vi "Unrock_Cluster_To_Unrock_Data.vi"(0 "Unrock_Cluster":T2, 1 "NAM":string, 2 "TDN":string, 3 "PROD":string, 4 "CALD":string, 5 "REV":string) -> (17 "Cluster67":T1)   [LabVIEW 2019]
uses:
  Unrock_Cluster.ctl
  Test_load.ctl
  Hardness_test.ctl
  Unrock_Data.ctl
  TEST.lvclass
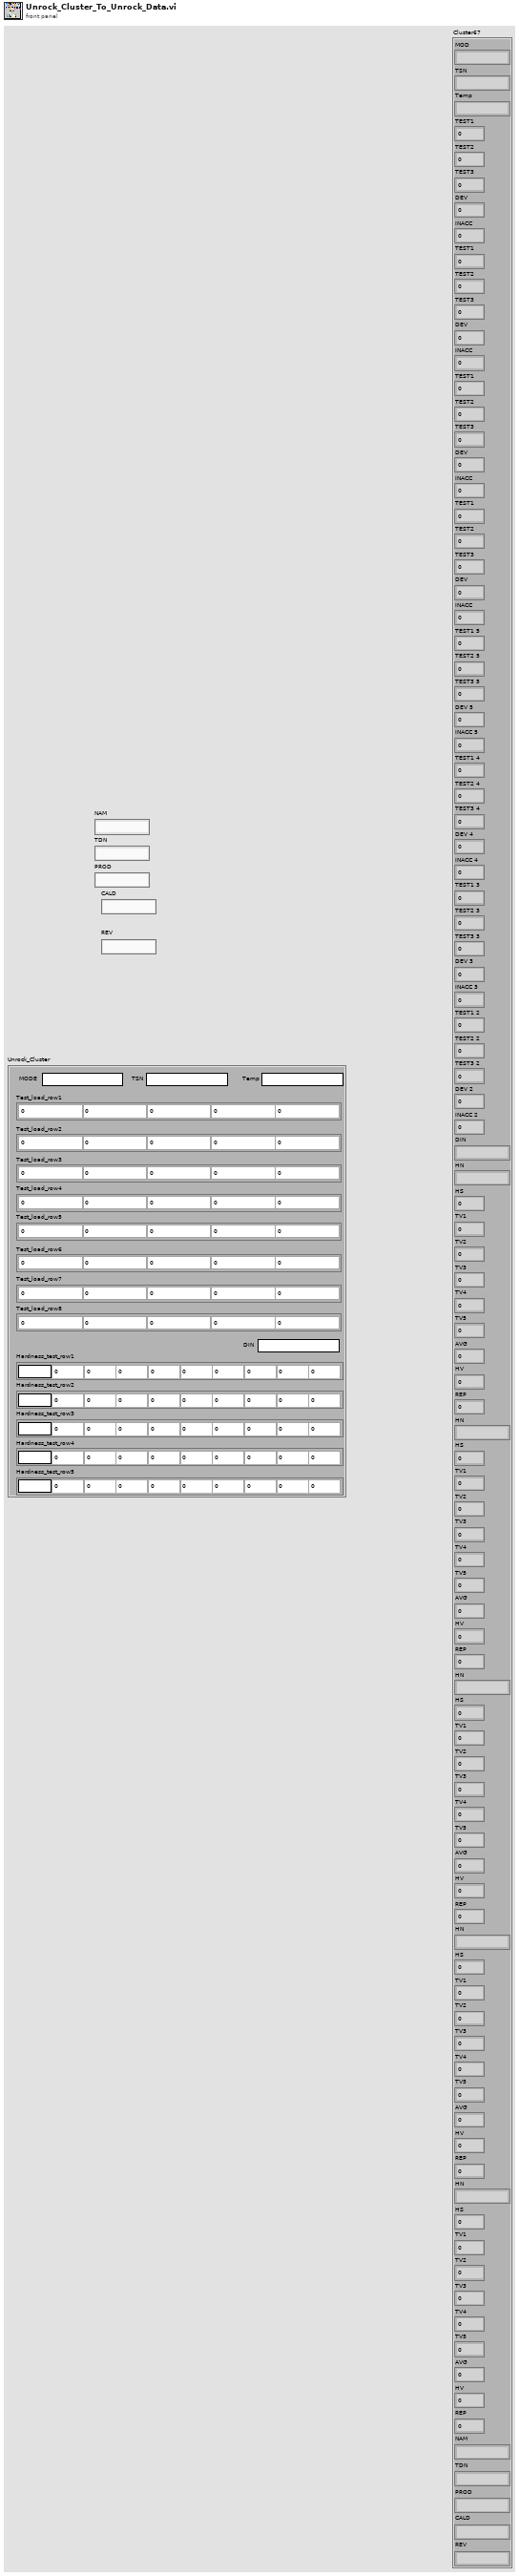
[diagram p1: front panel]
types:
  T1 = typedef "TEST.lvclass/Unrock_Data.ctl" = cluster{"MOD":string, "TSN":string, "Temp":string, "TEST1":sgl, "TEST2":sgl, "TEST3":sgl, "DEV":sgl, "INACC":sgl, "TEST1":sgl, "TEST2":sgl, "TEST3":sgl, "DEV":sgl, "INACC":sgl, "TEST1":sgl, "TEST2":sgl, "TEST3":sgl, "DEV":sgl, "INACC":sgl, "TEST1":sgl, "TEST2":sgl, "TEST3":sgl, "DEV":sgl, "INACC":sgl, "TEST1 5":sgl, "TEST2 5":sgl, "TEST3 5":sgl, "DEV 5":sgl, "INACC 5":sgl, "TEST1 4":sgl, "TEST2 4":sgl, "TEST3 4":sgl, "DEV 4":sgl, "INACC 4":sgl, "TEST1 3":sgl, "TEST2 3":sgl, "TEST3 3":sgl, "DEV 3":sgl, "INACC 3":sgl, "TEST1 2":sgl, "TEST2 2":sgl, "TEST3 2":sgl, "DEV 2":sgl, "INACC 2":sgl, "DIN":string, "HN":string, "HS":sgl, "TV1":sgl, "TV2":sgl, "TV3":sgl, "TV4":sgl, "TV5":sgl, "AVG":sgl, "HV":sgl, "REP":sgl, "HN":string, "HS":sgl, "TV1":sgl, "TV2":sgl, "TV3":sgl, "TV4":sgl, "TV5":sgl, "AVG":sgl, "HV":sgl, "REP":sgl, "HN":string, "HS":sgl, "TV1":sgl, "TV2":sgl, "TV3":sgl, "TV4":sgl, "TV5":sgl, "AVG":sgl, "HV":sgl, "REP":sgl, "HN":string, "HS":sgl, "TV1":sgl, "TV2":sgl, "TV3":sgl, "TV4":sgl, "TV5":sgl, "AVG":sgl, "HV":sgl, "REP":sgl, "HN":string, "HS":sgl, "TV1":sgl, "TV2":sgl, "TV3":sgl, "TV4":sgl, "TV5":sgl, "AVG":sgl, "HV":sgl, "REP":sgl, "NAM":string, "TDN":string, "PROD":string, "CALD":string, "REV":string}
  T2 = typedef "TEST.lvclass/Unrock_Cluster.ctl" = cluster{"MODE":string, "TSN":string, "Temp":string, "Test_load_row1":T3, "Test_load_row2":T3, "Test_load_row3":T3, "Test_load_row4":T3, "Test_load_row5":T3, "Test_load_row6":T3, "Test_load_row7":T3, "Test_load_row8":T3, "DIN":string, "Hardness_test_row1":T4, "Hardness_test_row2":T4, "Hardness_test_row3":T4, "Hardness_test_row4":T4, "Hardness_test_row5":T4}
  T3 = typedef "TEST.lvclass/Test_load.ctl" = cluster{"TEST1":sgl, "TEST2":sgl, "TEST3":sgl, "DEV":sgl, "INACC":sgl}
  T4 = typedef "TEST.lvclass/Hardness_test.ctl" = cluster{"HN":string, "HS":sgl, "TV1":sgl, "TV2":sgl, "TV3":sgl, "TV4":sgl, "TV5":sgl, "AVG":sgl, "HV":sgl, "REP":sgl}
  T5 = cluster{"MODE":string, "TSN":string, "Temp":string, "TEST1":sgl, "TEST2":sgl, "TEST3":sgl, "DEV":sgl, "INACC":sgl, "TEST1":sgl, "TEST2":sgl, "TEST3":sgl, "DEV":sgl, "INACC":sgl, "TEST1":sgl, "TEST2":sgl, "TEST3":sgl, "DEV":sgl, "INACC":sgl, "TEST1":sgl, "TEST2":sgl, "TEST3":sgl, "DEV":sgl, "INACC":sgl, "TEST1":sgl, "TEST2":sgl, "TEST3":sgl, "DEV":sgl, "INACC":sgl, "TEST1":sgl, "TEST2":sgl, "TEST3":sgl, "DEV":sgl, "INACC":sgl, "TEST1":sgl, "TEST2":sgl, "TEST3":sgl, "DEV":sgl, "INACC":sgl, "TEST1":sgl, "TEST2":sgl, "TEST3":sgl, "DEV":sgl, "INACC":sgl, "DIN":string, "HN":string, "HS":sgl, "TV1":sgl, "TV2":sgl, "TV3":sgl, "TV4":sgl, "TV5":sgl, "AVG":sgl, "HV":sgl, "REP":sgl, "HN":string, "HS":sgl, "TV1":sgl, "TV2":sgl, "TV3":sgl, "TV4":sgl, "TV5":sgl, "AVG":sgl, "HV":sgl, "REP":sgl, "HN":string, "HS":sgl, "TV1":sgl, "TV2":sgl, "TV3":sgl, "TV4":sgl, "TV5":sgl, "AVG":sgl, "HV":sgl, "REP":sgl, "HN":string, "HS":sgl, "TV1":sgl, "TV2":sgl, "TV3":sgl, "TV4":sgl, "TV5":sgl, "AVG":sgl, "HV":sgl, "REP":sgl, "HN":string, "HS":sgl, "TV1":sgl, "TV2":sgl, "TV3":sgl, "TV4":sgl, "TV5":sgl, "AVG":sgl, "HV":sgl, "REP":sgl, "NAM":string, "TDN":string, "PROD":string, "CALD":string, "REV":string}
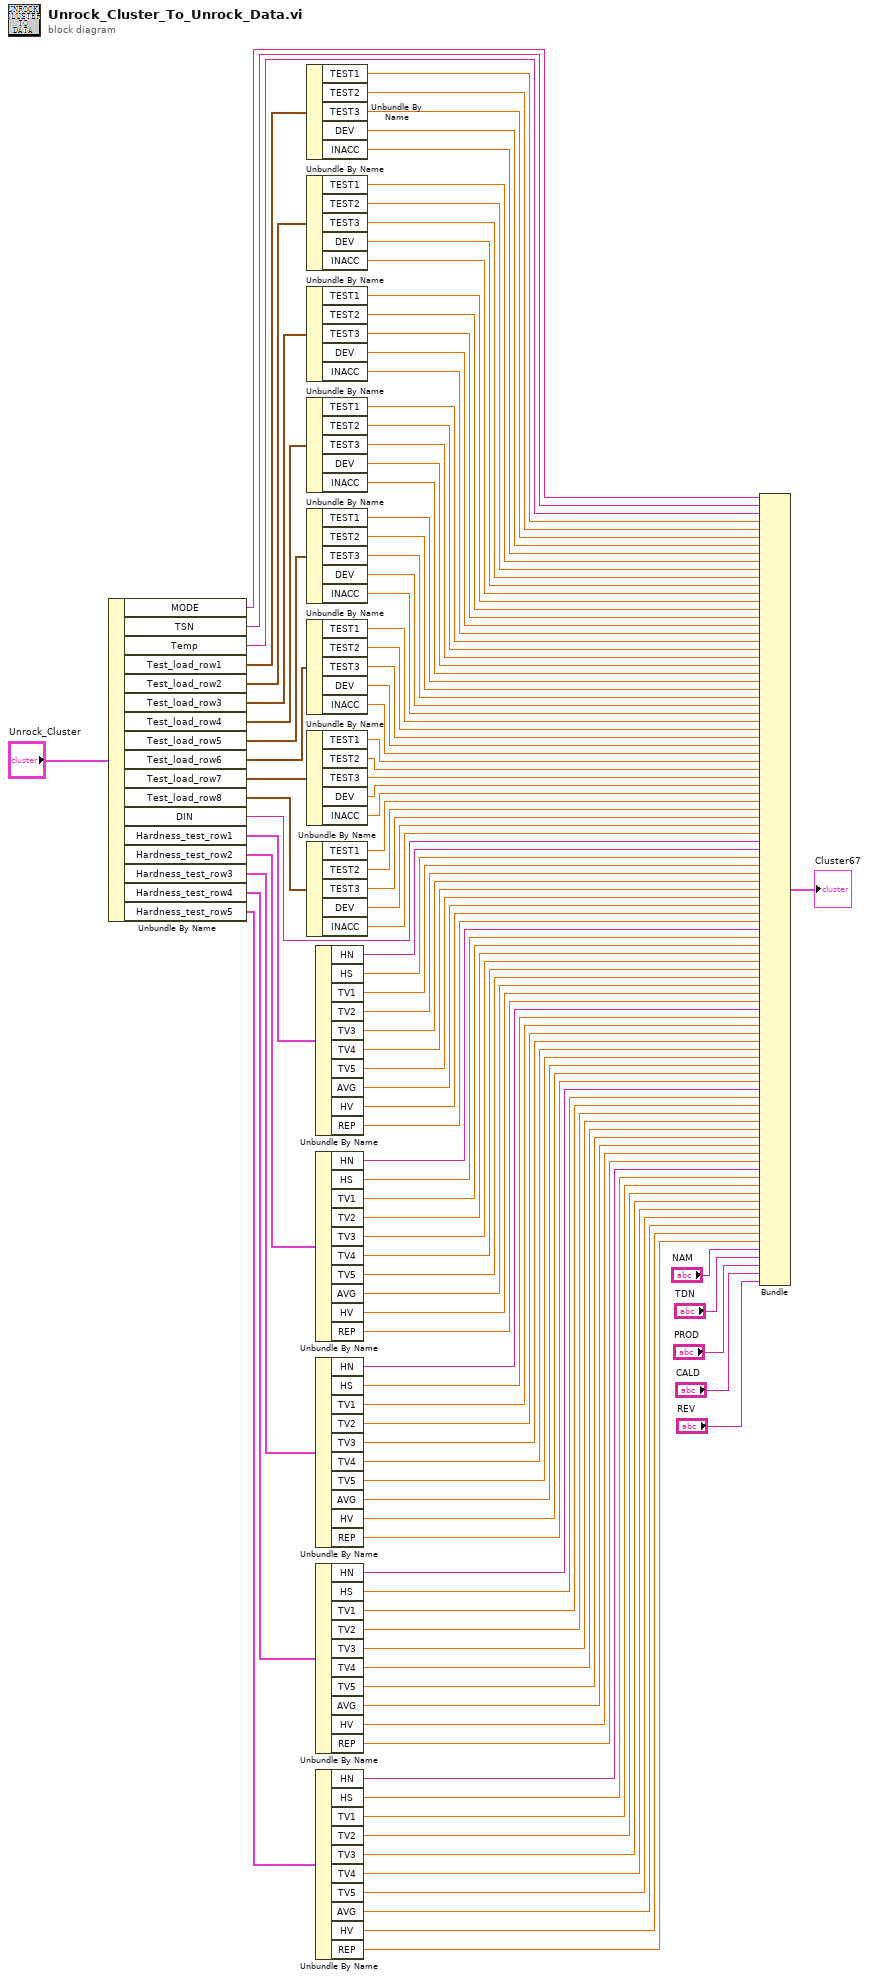
[diagram p0: block diagram]
diagram:
  n1 = Unbundle By Name("Unrock_Cluster") -> ("MODE"=w7:string, "TSN"=w8:string, "Temp"=w9:string, "Test_load_row1"=w57:T3, "Test_load_row2"=w56:T3, "Test_load_row3"=w55:T3, "Test_load_row4"=w54:T3, "Test_load_row5"=w53:T3, "Test_load_row6"=w52:T3, "Test_load_row7"=w51:T3, "Test_load_row8"=w50:T3, "DIN"=w59:string, "Hardness_test_row1"=w65:T4, "Hardness_test_row2"=w64:T4, "Hardness_test_row3"=w63:T4, "Hardness_test_row4"=w62:T4, "Hardness_test_row5"=w61:T4)
  n2 = Unbundle By Name(w57) -> ("TEST1"=w10:sgl, "TEST2"=w11:sgl, "TEST3"=w12:sgl, "DEV"=w13:sgl, "INACC"=w14:sgl)
  n3 = Unbundle By Name(w56) -> ("TEST1"=w15:sgl, "TEST2"=w16:sgl, "TEST3"=w17:sgl, "DEV"=w18:sgl, "INACC"=w19:sgl)
  n4 = Unbundle By Name(w55) -> ("TEST1"=w20:sgl, "TEST2"=w21:sgl, "TEST3"=w22:sgl, "DEV"=w23:sgl, "INACC"=w24:sgl)
  n5 = Unbundle By Name(w54) -> ("TEST1"=w25:sgl, "TEST2"=w26:sgl, "TEST3"=w27:sgl, "DEV"=w28:sgl, "INACC"=w29:sgl)
  n6 = Unbundle By Name(w53) -> ("TEST1"=w30:sgl, "TEST2"=w31:sgl, "TEST3"=w32:sgl, "DEV"=w33:sgl, "INACC"=w34:sgl)
  n7 = Unbundle By Name(w52) -> ("TEST1"=w35:sgl, "TEST2"=w36:sgl, "TEST3"=w37:sgl, "DEV"=w38:sgl, "INACC"=w39:sgl)
  n8 = Unbundle By Name(w51) -> ("TEST1"=w40:sgl, "TEST2"=w41:sgl, "TEST3"=w42:sgl, "DEV"=w43:sgl, "INACC"=w44:sgl)
  n9 = Unbundle By Name(w50) -> ("TEST1"=w45:sgl, "TEST2"=w46:sgl, "TEST3"=w47:sgl, "DEV"=w48:sgl, "INACC"=w49:sgl)
  n10 = Unbundle By Name(w65) -> ("HN"=w60:string, "HS"=w114:sgl, "TV1"=w113:sgl, "TV2"=w112:sgl, "TV3"=w111:sgl, "TV4"=w110:sgl, "TV5"=w109:sgl, "AVG"=w108:sgl, "HV"=w107:sgl, "REP"=w106:sgl)
  n11 = Unbundle By Name(w64) -> ("HN"=w105:string, "HS"=w104:sgl, "TV1"=w103:sgl, "TV2"=w102:sgl, "TV3"=w101:sgl, "TV4"=w100:sgl, "TV5"=w99:sgl, "AVG"=w98:sgl, "HV"=w97:sgl, "REP"=w96:sgl)
  n12 = Unbundle By Name(w63) -> ("HN"=w95:string, "HS"=w94:sgl, "TV1"=w93:sgl, "TV2"=w92:sgl, "TV3"=w91:sgl, "TV4"=w90:sgl, "TV5"=w89:sgl, "AVG"=w88:sgl, "HV"=w87:sgl, "REP"=w86:sgl)
  n13 = Unbundle By Name(w62) -> ("HN"=w85:string, "HS"=w84:sgl, "TV1"=w83:sgl, "TV2"=w82:sgl, "TV3"=w81:sgl, "TV4"=w80:sgl, "TV5"=w79:sgl, "AVG"=w78:sgl, "HV"=w77:sgl, "REP"=w76:sgl)
  n14 = Unbundle By Name(w61) -> ("HN"=w75:string, "HS"=w74:sgl, "TV1"=w73:sgl, "TV2"=w72:sgl, "TV3"=w71:sgl, "TV4"=w70:sgl, "TV5"=w69:sgl, "AVG"=w68:sgl, "HV"=w67:sgl, "REP"=w66:sgl)
  n15 = Bundle("MODE"=w7, "TSN"=w8, "Temp"=w9, "TEST1"=w10, "TEST2"=w11, "TEST3"=w12, "DEV"=w13, "INACC"=w14, "TEST1"=w15, "TEST2"=w16, "TEST3"=w17, "DEV"=w18, "INACC"=w19, "TEST1"=w20, "TEST2"=w21, "TEST3"=w22, "DEV"=w23, "INACC"=w24, "TEST1"=w25, "TEST2"=w26, "TEST3"=w27, "DEV"=w28, "INACC"=w29, "TEST1"=w30, "TEST2"=w31, "TEST3"=w32, "DEV"=w33, "INACC"=w34, "TEST1"=w35, "TEST2"=w36, "TEST3"=w37, "DEV"=w38, "INACC"=w39, "TEST1"=w40, "TEST2"=w41, "TEST3"=w42, "DEV"=w43, "INACC"=w44, "TEST1"=w45, "TEST2"=w46, "TEST3"=w47, "DEV"=w48, "INACC"=w49, "DIN"=w59, "HN"=w60, "HS"=w114, "TV1"=w113, "TV2"=w112, "TV3"=w111, "TV4"=w110, "TV5"=w109, "AVG"=w108, "HV"=w107, "REP"=w106, "HN"=w105, "HS"=w104, "TV1"=w103, "TV2"=w102, "TV3"=w101, "TV4"=w100, "TV5"=w99, "AVG"=w98, "HV"=w97, "REP"=w96, "HN"=w95, "HS"=w94, "TV1"=w93, "TV2"=w92, "TV3"=w91, "TV4"=w90, "TV5"=w89, "AVG"=w88, "HV"=w87, "REP"=w86, "HN"=w85, "HS"=w84, "TV1"=w83, "TV2"=w82, "TV3"=w81, "TV4"=w80, "TV5"=w79, "AVG"=w78, "HV"=w77, "REP"=w76, "HN"=w75, "HS"=w74, "TV1"=w73, "TV2"=w72, "TV3"=w71, "TV4"=w70, "TV5"=w69, "AVG"=w68, "HV"=w67, "REP"=w66, "NAM"="NAM", "TDN"="TDN", "PROD"="PROD", "CALD"="CALD", "REV"="REV") -> (→"Cluster67":T5)  [unwired: 1 in]
